vi "Telescope Move to RA and DEC.vi"(8 "error in (no error)":errorcluster, 10 "Object out":T1, 11 "PRIME Telescope in":refnum<class "PRIME Telescope.lvclass">) -> (0 "error out":errorcluster, 3 "PRIME Telescope out":refnum<class "PRIME Telescope.lvclass">)   [LabVIEW 2024, in "PRIME Telescope.lvclass"]
uses:
  PRIME Telescope.lvclass
  typedefs/CC cluster Object.ctl
  typedefs/CC cluster sidereal rate.ctl
  typedefs/CC cluster RA and DEC.ctl
  typedefs/cc cluster muRA muDEC.ctl
  CC cluster Telescope Offsets.ctl
  Telescope cluster Equinox.ctl
  Telescope cluster Parallax.ctl
  Telescope cluster Rotator.ctl
  Telesope ring Frame.ctl
  PRIME Telescope.lvclass/PRIME Telescope.ctl
  Telescope.lvclass
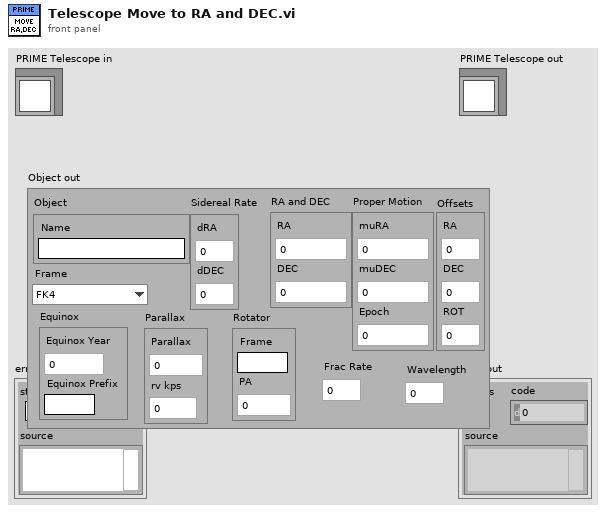
[diagram p1: front panel]
types:
  T1 = typedef "CC cluster Object.ctl" = cluster{"Object":cluster{"Name":string}, "Sidereal Rate":T2, "RA and DEC":T3, "Proper Motion":T4, "Offsets":T5, "Equinox":T6, "Parallax":T7, "Rotator":T8, "Frame":T9, "Frac Rate":dbl, "Wavelength":dbl}
  T2 = typedef "CC cluster sidereal rate.ctl" = cluster{"dRA":dbl, "dDEC":dbl}
  T3 = typedef "CC cluster RA and DEC.ctl" = cluster{"RA":dbl, "DEC":dbl}
  T4 = typedef "cc cluster muRA muDEC.ctl" = cluster{"muRA":dbl, "muDEC":dbl, "Epoch":dbl}
  T5 = typedef "CC cluster Telescope Offsets.ctl" = cluster{"RA":dbl, "DEC":dbl, "ROT":dbl}
  T6 = typedef "Telescope cluster Equinox.ctl" = cluster{"Equinox Year":i32, "Equinox Prefix":string}
  T7 = typedef "Telescope cluster Parallax.ctl" = cluster{"Parallax":dbl, "rv kps":dbl}
  T8 = typedef "Telescope cluster Rotator.ctl" = cluster{"Frame":string, "PA":dbl}
  T9 = typedef "Telesope ring Frame.ctl" = enum16{"FK4", "FK5", "APPT", "GAPPT", "AZEL"}
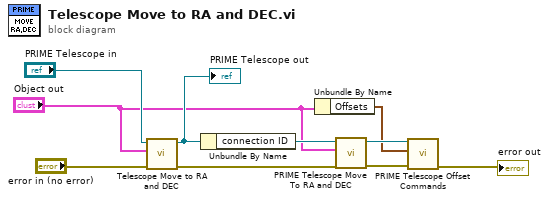
[diagram p0: block diagram]
diagram:
  n1 = call-parent "Telescope Move to RA and DEC.vi"("error in (no error)"="error in (no error)", "Object out"="Object out", "Telescope in"="PRIME Telescope in") -> ("error out"=w6:errorcluster, "Telescope out"=w8:refnum<class "PRIME Telescope.lvclass">)  [unwired: 7 in]
  "PRIME Telescope out" <- w8
  n2 = Unbundle By Name(w8) -> ("connection ID"=w7:refnum<k5>)
  n3 = Unbundle By Name("Object out") -> ("Offsets"=w1:T5)
  n4 = call "PRIME Telescope Move To RA and DEC.vi"("error in (no error)"=w6, "Object"="Object out", "connection ID"=w7) -> ("error out"=w5:errorcluster, "connection ID dup"=w3:refnum<k5>)  [unwired: 7 in]
  n5 = call "PRIME Telescope Offset Commands.vi"("error in (no error)"=w5, "Offsets"=w1, "connection ID"=w3) -> ("error out"=→"error out":errorcluster)  [unwired: 7 in, 1 out]
